vi "Test Permutate 3 chars.vi"(11 "Test Case In":refnum<class "Path Permutation Test.lvclass">) -> (0 "error out":errorcluster, 3 "Test Case Out":refnum<class "Path Permutation Test.lvclass">)   [LabVIEW 2020, in "Path Permutation Test.lvclass"]
uses:
  Path Permutation Test.lvclass
  C:/Program Files (x86)/National Instruments/LabVIEW 2020/vi.lib/Astemes/LUnit/Test Case.lvclass
  <vilib>/Astemes/LUnit/Test Case.lvclass/Test Case.ctl
  4993e8ee-a06a-463a-9684-69129f64d5ce.vi
  <vilib>/Astemes/LUnit/Append Pass Result.vi
  <vilib>/Astemes/LUnit/Append Fail Result.vi
  <vilib>/Astemes/LUnit/Describe Comparison.vi
  4993e8ee-a06a-463a-9684-69129f64d5ce.vi/9c5d11cd-9439-4240-a1ee-d9baace9c924.vi
  <vilib>/Astemes/LUnit/Run In UI.vi
  <vilib>/Utility/error.llb/Clear Errors.vi
  <vilib>/Astemes/LUnit/Describe Variant.vi
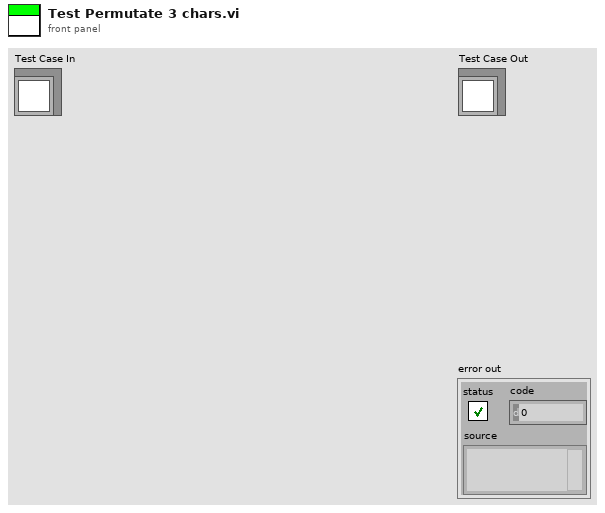
[diagram p1: front panel]
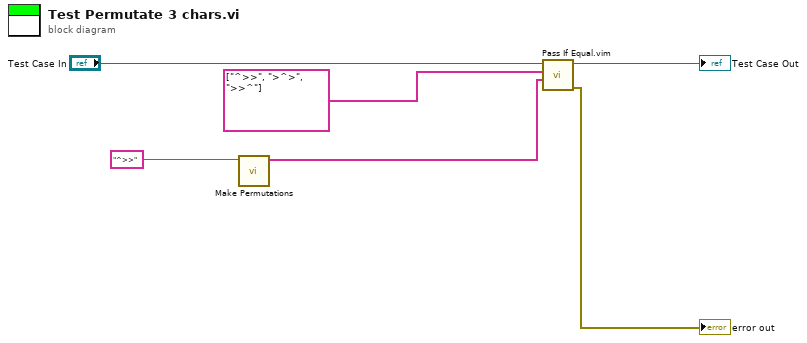
[diagram p0: block diagram]
diagram:
  n1 = call "Make Permutations.vi"("String"="^>>") -> ("Array"=w3:string[])  [unwired: 10 in]
  n2 = call "Pass If Equal.vim"("Actual"=w3, "Expected"=string[] ["^>>", ">^>", ">>^"], "LUnit Test Case In"="Test Case In") -> ("error out"=→"error out":errorcluster, "LUnit Test Case Out"=→"Test Case Out":refnum<class "Path Permutation Test.lvclass">)  [unwired: 7 in]
